vi "Action engine for shared variables.vi"(7 "read/write":enum16{"Read", "Write"}(ring), 10 "error in (no error)":errorcluster, 11 "func global variables write":T1={"Number of hours To Collect before starting new file "=1, "Base File Path"=path "", "Update setup"=TRUE, "Shutdown software"=TRUE, "Time between samples (seconds)"=5} {"Time between samples (seconds)" min=1 max=600 step=1; "Number of hours To Collect before starting new file" min=1 max=24 step=1}) -> (2 "error out":errorcluster, 3 "func global variables read":T1)   [LabVIEW 2011]
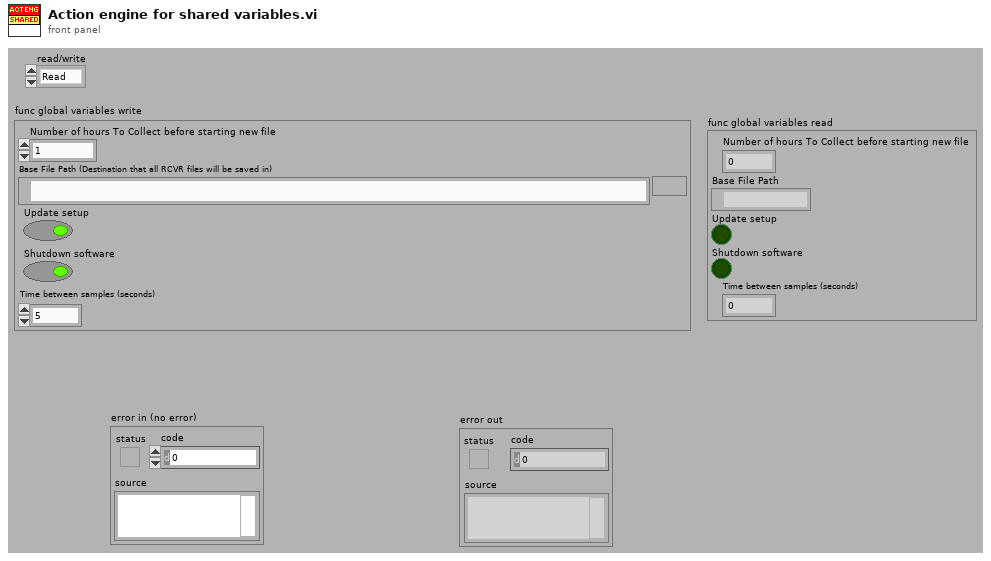
[diagram p1: front panel]
types:
  T1 = cluster{"Number of hours To Collect before starting new file ":u16, "Base File Path":path, "Update setup":bool, "Shutdown software":bool, "Time between samples (seconds)":u32}
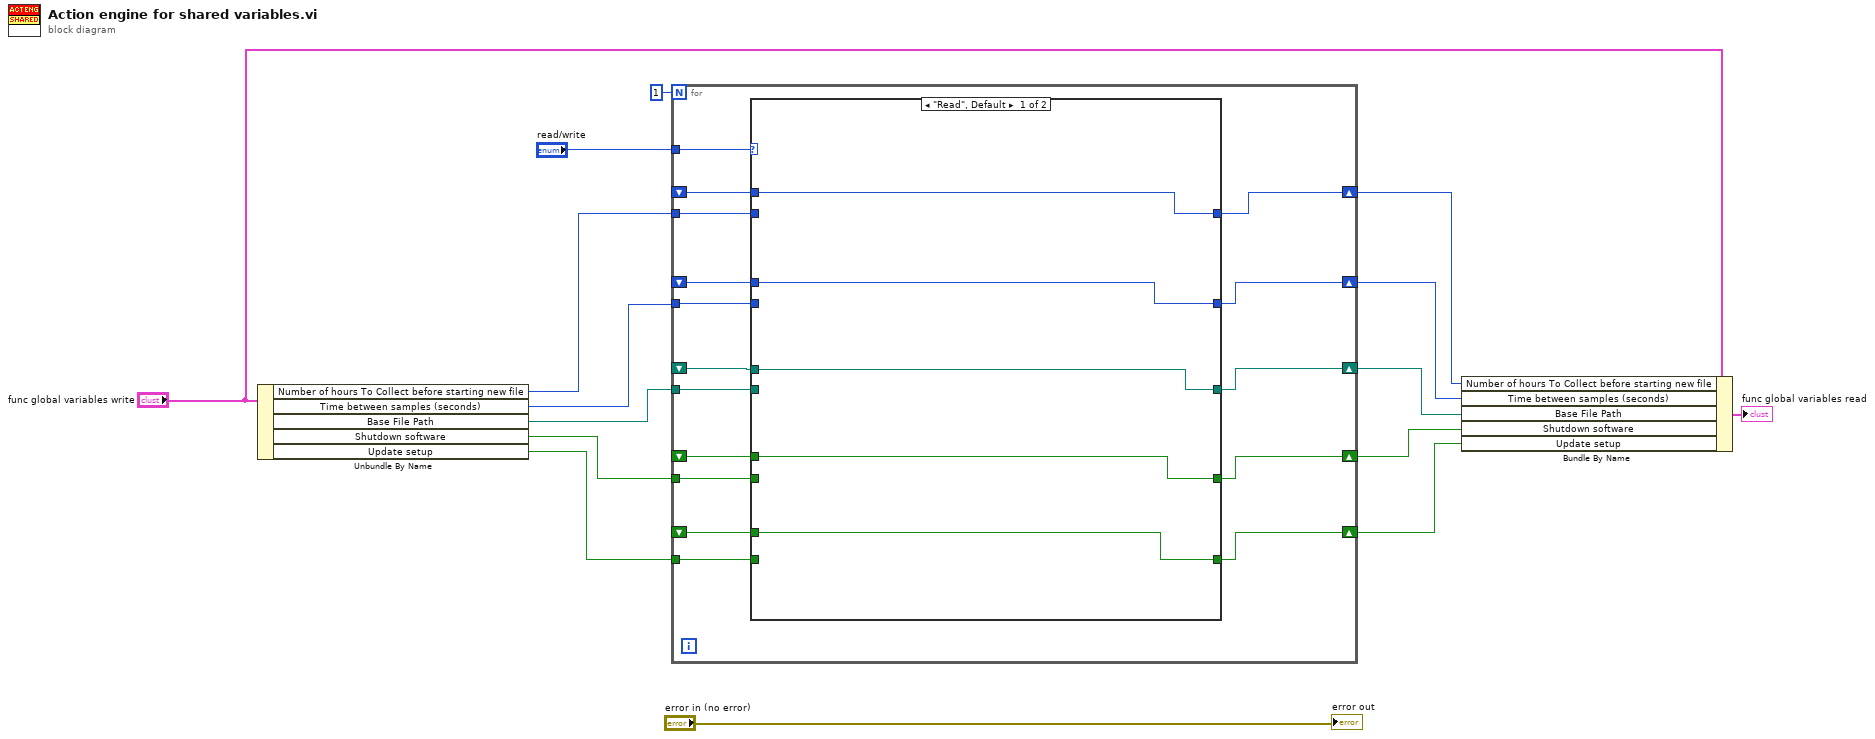
[diagram p0: block diagram]
diagram:
  n1 = Unbundle By Name("func global variables write") -> ("Number of hours To Collect before starting new file"=w13:u16, "Time between samples (seconds)"=w12:u32, "Base File Path"=w11:path, "Shutdown software"=w10:bool, "Update setup"=w9:bool)
  n2 = for {
    N: 1 -> [_]
    tunnel: "read/write" -> [w31]
    tunnel: w13 -> [w30]
    shift-right: [w29] -> w7
    shift-left: _ -> [w28]
    tunnel: w11 -> [w27]
    shift-right: [w26] -> w5
    shift-left: _ -> [w23]
    tunnel: w10 -> [w25]
    shift-right: [w24] -> w4
    shift-left: _ -> [w22]
    tunnel: w9 -> [w21]
    shift-right: [w20] -> w3
    shift-left: _ -> [w19]
    tunnel: w12 -> [w18]
    shift-right: [w17] -> w6
    shift-left: _ -> [w16]
    n3 = case shown="\"Read\", Default" w31 {
      tunnel: w30 -> [_ w41]
      tunnel: [w36 w41] -> w29
      tunnel: w28 -> [w36 _]
      tunnel: w27 -> [_ w40]
      tunnel: [w34 w40] -> w26
      tunnel: w25 -> [_ w39]
      tunnel: [w33 w39] -> w24
      tunnel: w23 -> [w34 _]
      tunnel: w22 -> [w33 _]
      tunnel: w21 -> [_ w38]
      tunnel: [w32 w38] -> w20
      tunnel: w19 -> [w32 _]
      tunnel: w18 -> [_ w37]
      tunnel: [w35 w37] -> w17
      tunnel: w16 -> [w35 _]
      frame "Read", Default {
      }
      frame "Write" {
      }
    }
  }
  n4 = Bundle By Name(cluster="func global variables write", "Number of hours To Collect before starting new file"=w7, "Time between samples (seconds)"=w6, "Base File Path"=w5, "Shutdown software"=w4, "Update setup"=w3) -> (→"func global variables read":T1)
  "error out" <- "error in (no error)"
